vi "UnZip Prime.vi"(8 "error in":errorcluster, 11 "Path":path=path "C:/Users/mw24/Documents/Final Designs - Prime/MasterProgram.mcdx") -> (0 "error out":errorcluster, 3 "Variable Clusters out":T1)   [LabVIEW 2011, in "Design Server.lvlib"]
uses:
  Design Server.lvlib
  Variable cluster.ctl
  <vilib>/zip/NI_Unzip.lvlib
panel:
  out "worksheet":string
  out "result":string
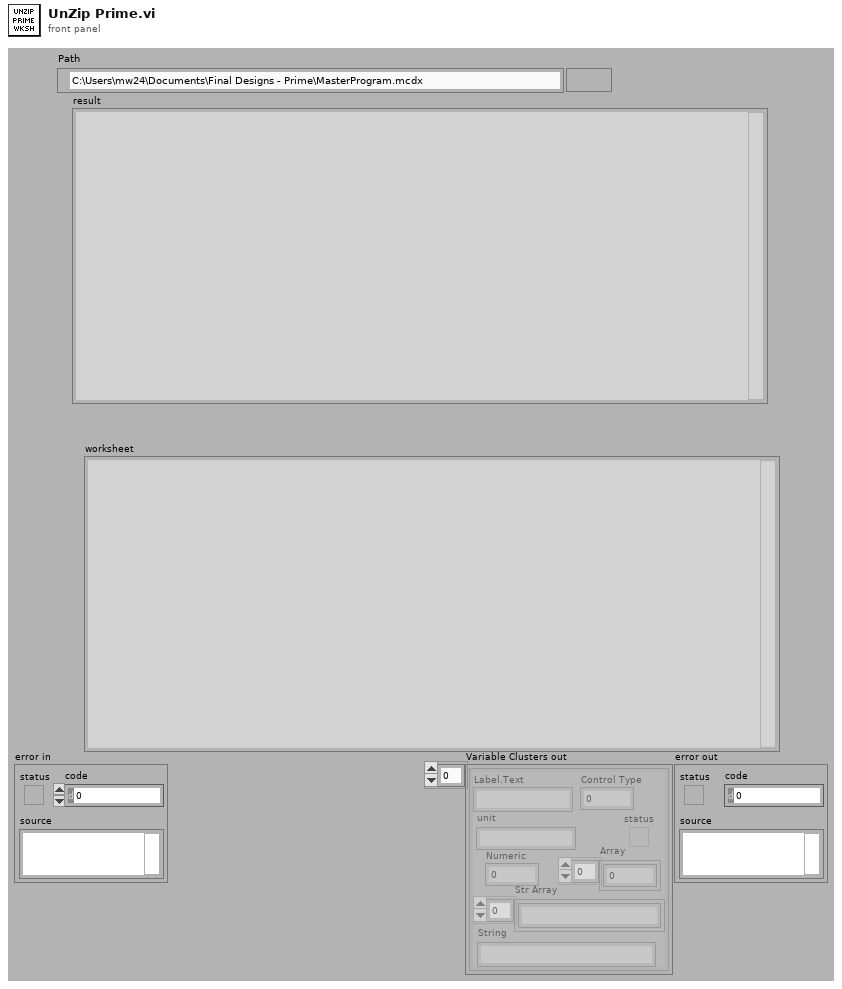
[diagram p1: front panel]
types:
  T1 = typedef "Design Server.lvlib/Variable cluster.ctl" = cluster{"Label.Text":string, "Control Type":u32, "Numeric":dbl, "Array":dbl[], "status":bool, "Str Array":string[], "String":string, "unit":string}[]
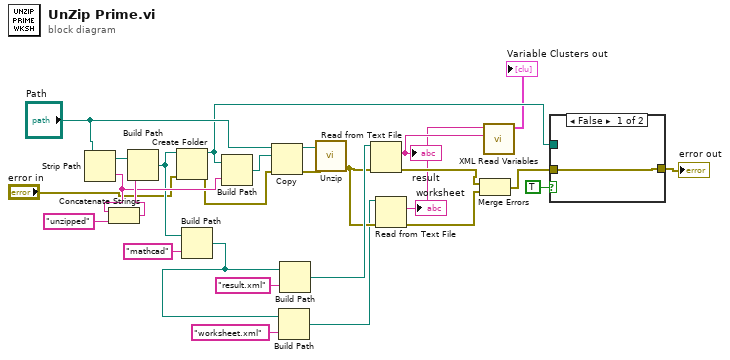
[diagram p0: block diagram]
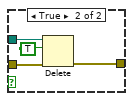
[diagram p2: hidden frame]
diagram:
  n1 = Strip Path(path="Path") -> (stripped path=w26:path, name=w22:string)
  n2 = Concatenate Strings(w22, "unzipped" ("name or relative path")) -> (w24:string)
  n3 = Build Path(base path=w26, name or relative path=w24) -> (appended path=w20:path)
  n4 = Create Folder(path (use dialog)=w20, error in="error in") -> (created path=w15:path, error out=w3:errorcluster)  [unwired: 1 in, 1 out]
  n5 = Build Path(base path=w20, name or relative path="mathcad") -> (appended path=w12:path)
  n6 = Build Path(base path=w15, name or relative path=w22) -> (appended path=w21:path)
  n7 = Copy(8:w3, 10:w21, 11:"Path") -> (0:w16:errorcluster, 3:w27:path)  [unwired: 2 in, 1 out]
  n8 = Build Path(base path=w12, name or relative path="worksheet.xml") -> (appended path=w10:path)
  n9 = Build Path(base path=w12, name or relative path="result.xml") -> (appended path=w17:path)
  n10 = call <vilib>:"Unzip.vi"("error in (no error)"=w16, "Zip file"=w27) -> ("error out"=w11:errorcluster)  [unwired: 7 in, 2 out]
  n11 = Read from Text File(file (use dialog)=w17, error in=w11) -> (text=w6:string, error out=w9:errorcluster)  [unwired: 2 in, 2 out]
  "result" <- w6
  n12 = Read from Text File(file (use dialog)=w10, error in=w11) -> (text=w5:string, error out=w8:errorcluster)  [unwired: 2 in, 2 out]
  "worksheet" <- w5
  n13 = Merge Errors(w9, w8) -> (w7:errorcluster)
  n14 = call "XML Read Variables.vi"("XML Result"=w6, "XML Worksheet"=w5) -> ("Variable Clusters out"=→"Variable Clusters out":T1)  [unwired: 9 in]
  n15 = case shown="False" TRUE {
    tunnel: w7 -> [w28 w32]
    tunnel: w15 -> [_ w31]
    tunnel: [w28 w29] -> w1
    frame False {
    }
    frame True {
      n16 = Delete(path (use dialog)=w31, entire hierarchy (F)=TRUE, error in=w32) -> (error out=w29:errorcluster)  [unwired: 2 in, 2 out]
    }
  }
  "error out" <- w1
